vi "Start Measurement.vi"(8 "error in (no error)":errorcluster, 11 "Cap Bank Idot Measurement in":refnum<class "Cap Bank Idot Measurement.lvclass">) -> (0 "error out":errorcluster, 3 "Cap Bank Idot Measurement out":refnum<class "Cap Bank Idot Measurement.lvclass">)   [LabVIEW 2012]
uses:
  NI-DAQ/Mag Lab Measure/DAQmx Digitizer/DAQmx Digitizer.lvclass
  <vilib>/ActorFramework/Actor/Actor.lvclass
  Mag Lab Measure Controller Messages/Log Status Update Msg/Log Status Update Msg.lvclass
  Cap Bank Idot Measurement.lvclass
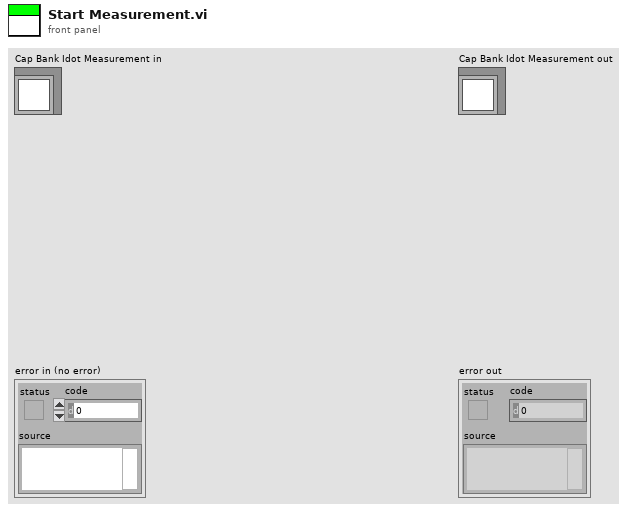
[diagram p1: front panel]
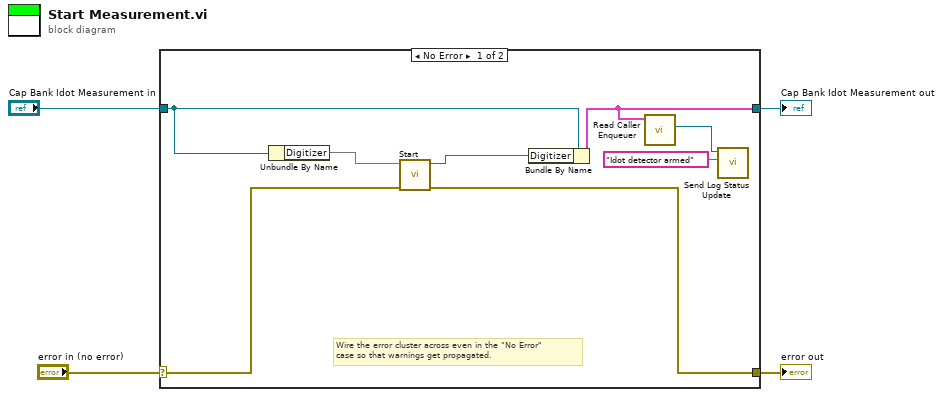
[diagram p0: block diagram]
diagram:
  n1 = case shown="No Error" "error in (no error)" {
    selector: "error in (no error)" -> [w9 w14]
    tunnel: [w8 w14] -> w3
    tunnel: [w7 w13] -> w1
    tunnel: "Cap Bank Idot Measurement in" -> [w12 w13]
    frame No Error {
      # "Wire the error cluster across even in the \"No Error\"\ncase so that warnings get propagated."
      n2 = Unbundle By Name(w12) -> ("Digitizer"=w11)
      n3 = call-dynamic "Start.vi"("error in (no error)"=w9, "DAQmx Digitizer in"=w11) -> ("error out"=w8:errorcluster, "DAQmx Digitizer out"=w10:refnum<class "DAQmx Digitizer.lvclass">)  [unwired: 8 in]
      n4 = Bundle By Name(cluster=w12, "Digitizer"=w10) -> (w7:cluster{})
      n5 = call <vilib>:"Read Caller Enqueuer.vi"("Actor"=w7) -> ("Caller Enqueuer"=w5:refnum<class "Message Enqueuer.lvclass">)  [unwired: 10 in]
      n6 = call "Send Log Status Update.vi"("Status"="Idot detector armed", "Message Enqueuer"=w5) -> ()  [unwired: 8 in, 2 out]
    }
    frame Error {
    }
  }
  "error out" <- w3
  "Cap Bank Idot Measurement out" <- w1
